vi "Group_Project-REV7.vi"() -> ()   [LabVIEW 2022 SP3]
uses:
  Control 1.ctl
panel:
  out "Train Waiting":bool=TRUE
  out "Boolean":bool=TRUE
  out "Numeric":i32
  out "Train go which way":dbl
  out "Increment Slider":bool=TRUE
  out "Timestamp for slide":i32
  out "Time stamp for wait":i32
  out "Ready for train":bool
  out "Train Progress":dbl(slide) scale=0.0..100.0
  out "Train Nearby Sensor 2":bool
  out "Train Nearby Sensor 1":bool
  out "Wait Time":i32
  out "Traffic Count":i32
  out "Observe traffic":bool
  out "Busy traffic":bool
  out "Add wait time":i32
  out "Numeric 5":u32
  out "Cars to Stop":bool
  out "Numeric 4":u32
  out "Car To Go":bool
  out "Train?":bool
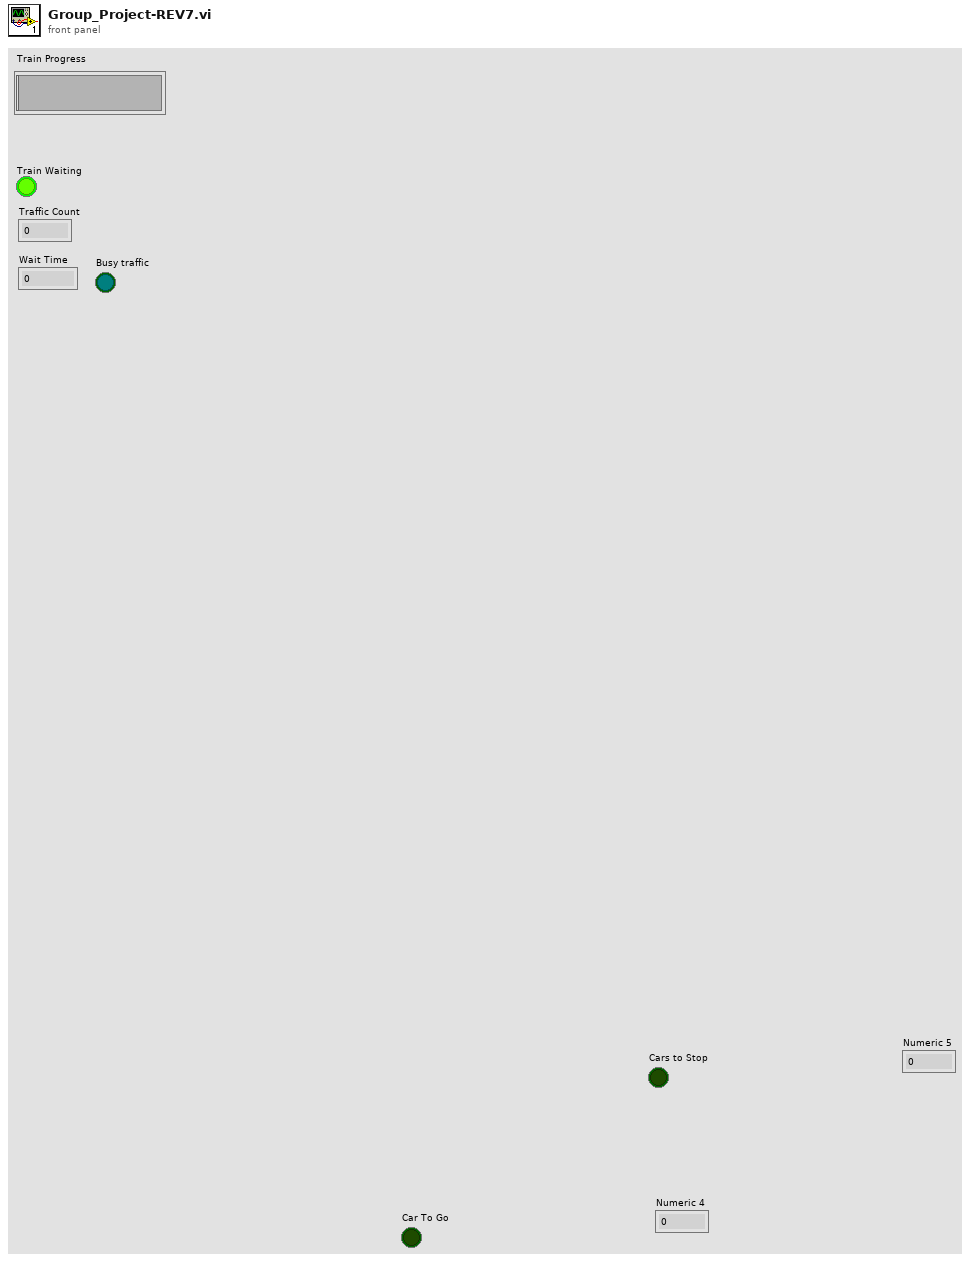
[diagram p1: front panel]
types:
  T1 = typedef "Control 1.ctl" = enum16{"None", "Down", "Up"}
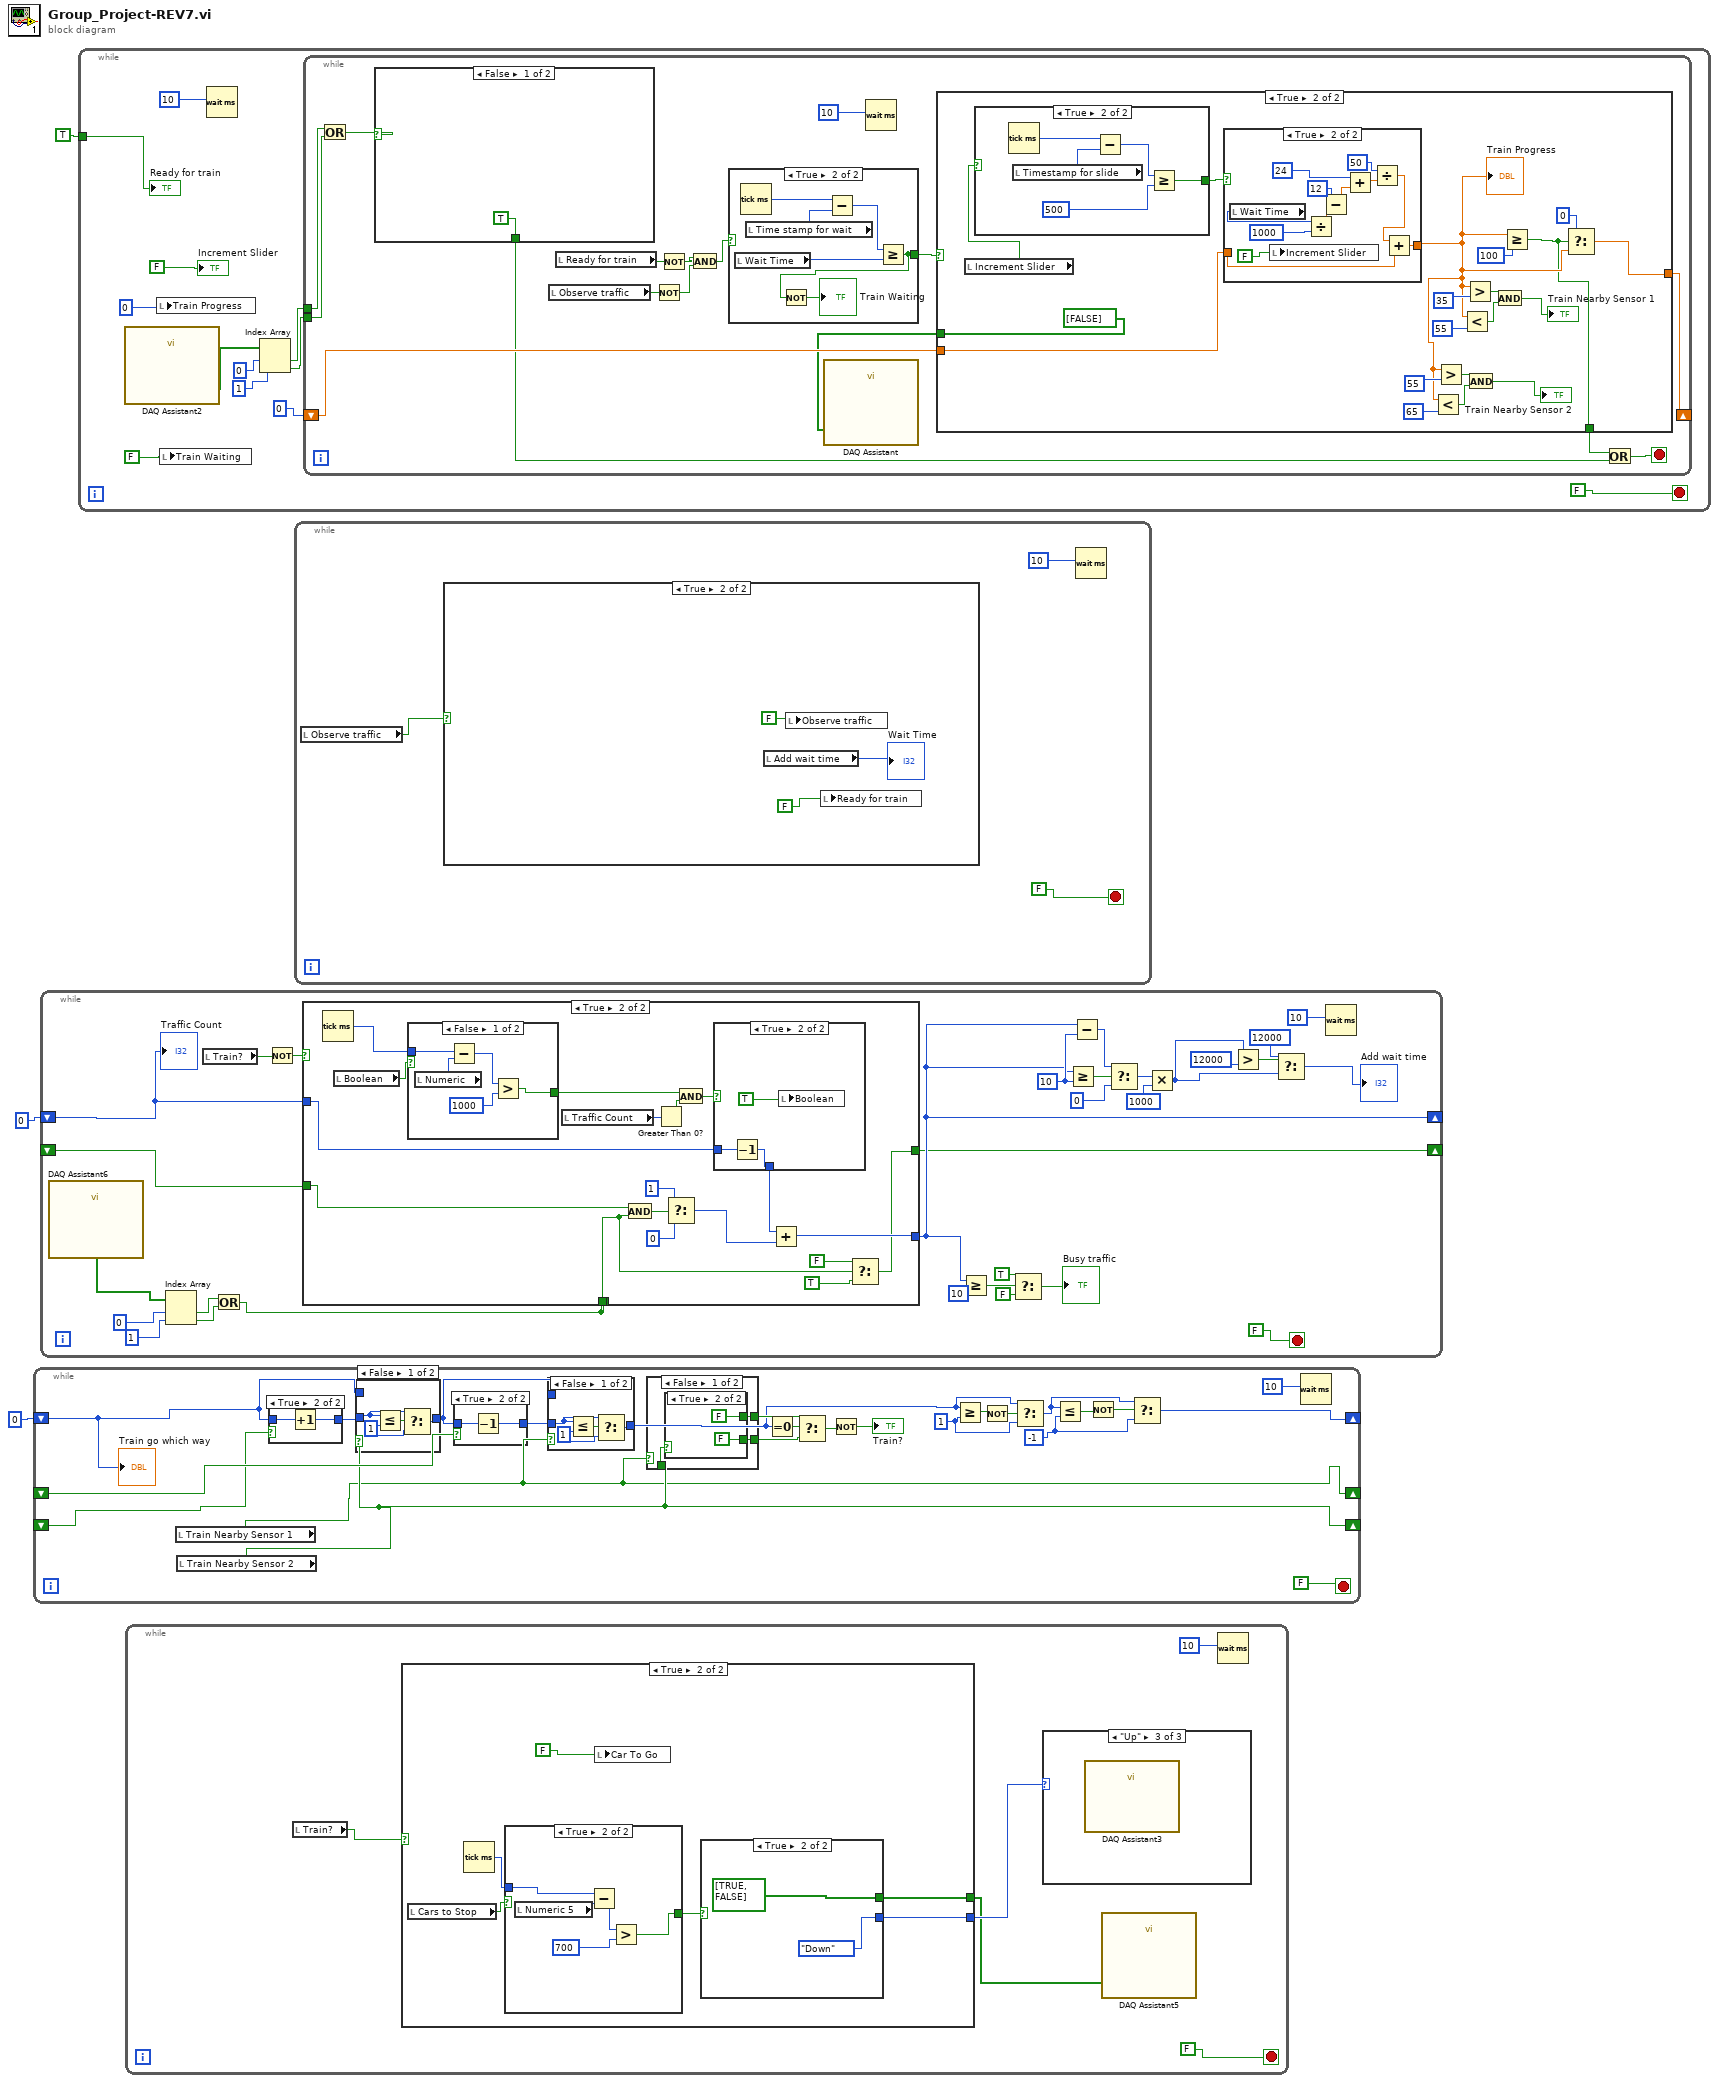
[diagram p0: block diagram]
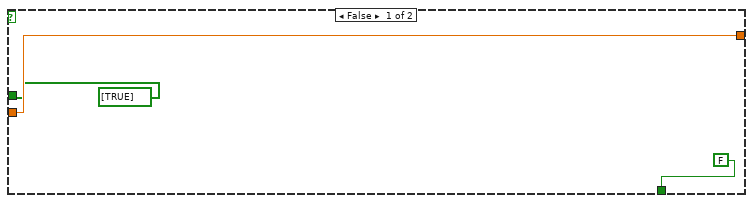
[diagram p3: hidden frame]
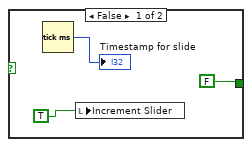
[diagram p5: hidden frame]
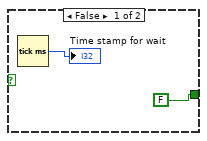
[diagram p6: hidden frame]
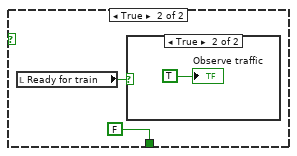
[diagram p7: hidden frame]
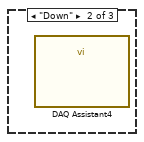
[diagram p10: hidden frame]
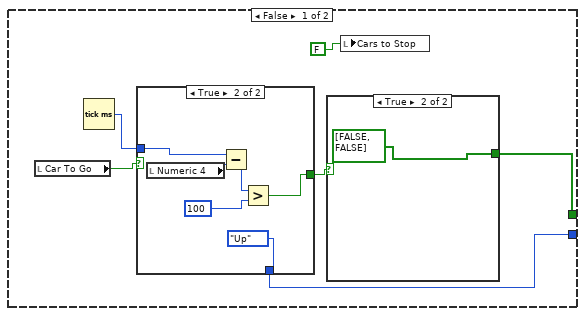
[diagram p11: hidden frame]
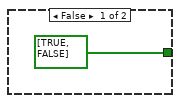
[diagram p12: hidden frame]
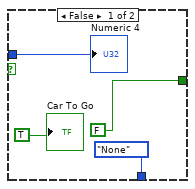
[diagram p13: hidden frame]
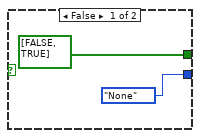
[diagram p14: hidden frame]
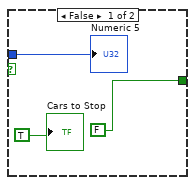
[diagram p15: hidden frame]
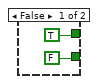
[diagram p16: hidden frame]
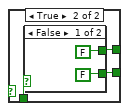
[diagram p17: hidden frame]
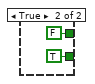
[diagram p18: hidden frame]
diagram:
  n1 = while {
    shift-right: [w8] -> _
    shift-left: 0 -> [w4]
    shift-right: [w6] -> _
    shift-left: _ -> [w10]
    shift-right: [w5] -> _
    shift-left: _ -> [w11]
    stop <- FALSE stop-if-true
    w14 = -1
    w17 = 1
    n2 = local read "Train Nearby Sensor 1"() -> (w5:bool)
    n3 = local read "Train Nearby Sensor 2"() -> (w6:bool)
    n4 = case shown="True" w10 {
      tunnel: [w55 w57] -> w27
      tunnel: w4 -> [w55 w56]
      frame False {
      }
      frame True {
        n5 = Increment(x=w56) -> (x+1=w57:i32)
      }
    }
    n6 = case shown="False" w6 {
      tunnel: w27 -> [w52 _]
      tunnel: [w50 w54] -> w26
      tunnel: w4 -> [_ w54]
      frame False {
        w51 = 1
        n7 = Less Or Equal?(x=w52, y=w51) -> (x <= y?=w53:bool)
        n8 = Select(t=w52, s=w53, f=w51) -> (s? t:f=w50:i32)
      }
      frame True {
      }
    }
    n9 = case shown="True" w11 {
      tunnel: w26 -> [w47 w49]
      tunnel: [w47 w48] -> w25
      frame False {
      }
      frame True {
        n10 = Decrement(x=w49) -> (x-1=w48:i32)
      }
    }
    n11 = case shown="False" w5 {
      tunnel: w26 -> [_ w46]
      tunnel: w25 -> [w43 _]
      tunnel: [w42 w46] -> w18
      frame False {
        w44 = 1
        n12 = Less Or Equal?(x=w43, y=w44) -> (x <= y?=w45:bool)
        n13 = Select(t=w43, s=w45, f=w44) -> (s? t:f=w42:i32)
      }
      frame True {
      }
    }
    n14 = case shown="False" w5 {
      tunnel: w6 -> [w28 w37]
      tunnel: [w29 w35] -> w23
      tunnel: [w30 w36] -> w22
      frame False {
        n15 = case shown="True" w28 {
          tunnel: [TRUE FALSE] -> w29
          tunnel: [FALSE FALSE] -> w30
          frame False {
          }
          frame True {
          }
        }
      }
      frame True {
        n16 = case shown="False" w37 {
          tunnel: [FALSE FALSE] -> w35
          tunnel: [FALSE TRUE] -> w36
          frame False {
          }
          frame True {
          }
        }
      }
    }
    n17 = Equal To 0?(x=w18) -> (x = 0?=w24:bool)
    n18 = Select(t=w23, s=w24, f=w22) -> (s? t:f=w21:bool)
    n19 = Not(x=w21) -> (.not. x?=→"Train?":bool)
    n20 = Greater Or Equal?(x=w18, y=w17) -> (x >= y?=w19:bool)
    n21 = Not(x=w19) -> (.not. x?=w20:bool)
    n22 = Select(t=w18, s=w20, f=w17) -> (s? t:f=w13:i32)
    n23 = Less Or Equal?(x=w13, y=w14) -> (x <= y?=w16:bool)
    n24 = Not(x=w16) -> (.not. x?=w15:bool)
    n25 = Select(t=w13, s=w15, f=w14) -> (s? t:f=w8:i32)
    n26 = Wait (ms)(milliseconds to wait=10) -> ()  [unwired: 1 out]
    "Train go which way" <- w4
  }
  n27 = while {
    shift-right: [w60] -> _
    shift-left: 0 -> [w62]
    shift-right: [w59] -> _
    shift-left: _ -> [w61]
    stop <- FALSE stop-if-true
    w85 = 10
    n28 = call "DAQ Assistant6"() -> ("data"=w69:bool[])  [unwired: 17 in, 2 out]
    n29 = Index Array(array=w69, index #1=0, index #2=1) -> (element #1=w66:bool, element #2=w65:bool)
    n30 = local read "Train?"() -> (w64:bool)
    n31 = Or(x=w66, y=w65) -> (x .or. y?=w58:bool)
    n32 = Not(x=w64) -> (.not. x?=w63:bool)
    n33 = case shown="True" w63 {
      tunnel: w62 -> [w92 w110]
      tunnel: w61 -> [w88 w106]
      tunnel: [w91 w104] -> w60
      tunnel: [w90 w101] -> w59
      tunnel: w58 -> [w89 _]
      tunnel: w58 -> [_ w100]
      frame False {
        n34 = And(x=w88, y=w89) -> (x .and. y?=w98:bool)
        n35 = Select(t=1, s=w98, f=0) -> (s? t:f=w95:i32)
        n36 = Add(x=w92, y=w95) -> (x+y=w91:i32)
        n37 = Select(t=FALSE, s=w89, f=TRUE) -> (s? t:f=w90:bool)
      }
      frame True {
        n38 = Tick Count (ms)() -> (millisecond timer value=w116:u32)
        n39 = local read "Boolean"() -> (w115:bool)
        n40 = case shown="False" w115 {
          tunnel: w116 -> [w124 w127]
          tunnel: [w121 w126] -> w114
          frame False {
            n41 = local read "Numeric"() -> (w125:i32)
            n42 = Subtract(x=w124, y=w125) -> (x-y=w122:u32)
            n43 = Greater?(x=w122, y=1000) -> (0:w121:bool)
          }
          frame True {
            w126 = FALSE
            "Numeric" <- w127
            "Boolean" <- w126
          }
        }
        n44 = local read "Traffic Count"() -> (w113:i32)
        n45 = And(x=w106, y=w100) -> (x .and. y?=w109:bool)
        n46 = Greater Than 0?(x=w113) -> (x > 0?=w112:bool)
        n47 = Select(t=1, s=w109, f=0) -> (s? t:f=w105:i32)
        n48 = And(x=w114, y=w112) -> (x .and. y?=w111:bool)
        n49 = case shown="True" w111 {
          tunnel: w110 -> [w117 w119]
          tunnel: [w117 w120] -> w99
          frame False {
          }
          frame True {
            n50 = Decrement(x=w119) -> (x-1=w120:i32)
            n51 = local write "Boolean"(TRUE) -> ()
          }
        }
        n52 = Add(x=w99, y=w105) -> (x+y=w104:i32)
        n53 = Select(t=FALSE, s=w100, f=TRUE) -> (s? t:f=w101:bool)
      }
    }
    n54 = Greater Or Equal?(x=w60, y=10) -> (x >= y?=w79:bool)
    n55 = Select(t=TRUE, s=w79, f=FALSE) -> (s? t:f=→"Busy traffic":bool)
    n56 = Greater Or Equal?(x=w60, y=w85) -> (x >= y?=w86:bool)
    n57 = Subtract(x=w60, y=w85) -> (x-y=w84:i32)
    n58 = Select(t=w84, s=w86, f=0) -> (s? t:f=w82:i32)
    n59 = Multiply(x=w82, y=1000) -> (x*y=w72:i32)
    n60 = Greater?(x=w72, y=12000) -> (0:w73:bool)
    n61 = Select(t=12000, s=w73, f=w72) -> (s? t:f=→"Add wait time":i32)
    n62 = Wait (ms)(milliseconds to wait=10) -> ()  [unwired: 1 out]
    "Traffic Count" <- w62
  }
  n63 = while {
    tunnel: TRUE -> [w130]
    stop <- FALSE stop-if-true
    n64 = call "DAQ Assistant2"() -> ("data"=w135:bool[])  [unwired: 17 in, 2 out]
    n65 = local write "Train Progress"(0) -> ()
    n66 = local write "Train Waiting"(FALSE) -> ()
    n67 = Wait (ms)(milliseconds to wait=10) -> ()  [unwired: 1 out]
    n68 = Index Array(array=w135, index #1=0, index #2=1) -> (element #1=w132:bool, element #2=w131:bool)
    n69 = while {
      tunnel: w132 -> [w155]
      tunnel: w131 -> [w149]
      shift-right: [w147] -> _
      shift-left: 0 -> [w148]
      stop <- w142 stop-if-true
      n70 = Or(x=w155, y=w149) -> (x .or. y?=w154:bool)
      n71 = case shown="False" w154 {
        tunnel: [TRUE FALSE] -> w141
        frame False {
        }
        frame True {
          n72 = local read "Ready for train"() -> (w209:bool)
          n73 = case shown="True" w209 {
            frame False {
            }
            frame True {
              "Observe traffic" <- TRUE
            }
          }
        }
      }
      n74 = local read "Observe traffic"() -> (w153:bool)
      n75 = local read "Ready for train"() -> (w144:bool)
      n76 = Not(x=w153) -> (.not. x?=w152:bool)
      n77 = Not(x=w144) -> (.not. x?=w145:bool)
      n78 = And(x=w145, y=w152) -> (x .and. y?=w151:bool)
      n79 = case shown="True" w151 {
        tunnel: [FALSE w201] -> w150
        frame False {
          n80 = Tick Count (ms)() -> (millisecond timer value=→"Time stamp for wait":u32)
        }
        frame True {
          n81 = local read "Wait Time"() -> (w203:i32)
          n82 = Tick Count (ms)() -> (millisecond timer value=w205:u32)
          n83 = local read "Time stamp for wait"() -> (w206:i32)
          n84 = Subtract(x=w205, y=w206) -> (x-y=w204:u32)
          n85 = Greater Or Equal?(x=w204, y=w203) -> (x >= y?=w201:bool)
          n86 = Not(x=w201) -> (.not. x?=→"Train Waiting":bool)
        }
      }
      n87 = Wait (ms)(milliseconds to wait=10) -> ()  [unwired: 1 out]
      n88 = case shown="True" w150 {
        tunnel: w148 -> [w158 w175]
        tunnel: [w158 w164] -> w147
        tunnel: [FALSE w160] -> w143
        tunnel: [bool[] [TRUE] bool[] [FALSE]] -> w140
        frame False {
        }
        frame True {
          n89 = local read "Increment Slider"() -> (w177:bool)
          n90 = case shown="True" w177 {
            tunnel: [FALSE w194] -> w176
            frame False {
              n91 = Tick Count (ms)() -> (millisecond timer value=→"Timestamp for slide":u32)
              n92 = local write "Increment Slider"(TRUE) -> ()
            }
            frame True {
              n93 = Tick Count (ms)() -> (millisecond timer value=w198:u32)
              n94 = local read "Timestamp for slide"() -> (w197:i32)
              n95 = Subtract(x=w198, y=w197) -> (x-y=w196:u32)
              n96 = Greater Or Equal?(x=w196, y=500) -> (x >= y?=w194:bool)
            }
          }
          n97 = case shown="True" w176 {
            tunnel: w175 -> [w178 w184]
            tunnel: [w178 w183] -> w165
            frame False {
            }
            frame True {
              n98 = local read "Wait Time"() -> (w189:i32)
              n99 = local write "Increment Slider"(FALSE) -> ()
              n100 = Divide(x=w189, y=1000) -> (x/y=w181:dbl)
              n101 = Subtract(x=12, y=w181) -> (x-y=w179:dbl)
              n102 = Add(x=24, y=w179) -> (x+y=w186:dbl)
              n103 = Divide(x=50, y=w186) -> (x/y=w185:dbl)
              n104 = Add(x=w185, y=w184) -> (x+y=w183:dbl)
            }
          }
          "Train Progress" <- w165
          n105 = Less?(x=w165, y=65) -> (x < y?=w168:bool)
          n106 = Greater?(x=w165, y=55) -> (0:w169:bool)
          n107 = Less?(x=w165, y=55) -> (x < y?=w172:bool)
          n108 = Greater?(x=w165, y=35) -> (0:w173:bool)
          n109 = And(x=w169, y=w168) -> (x .and. y?=→"Train Nearby Sensor 2":bool)
          n110 = And(x=w173, y=w172) -> (x .and. y?=→"Train Nearby Sensor 1":bool)
          n111 = Greater Or Equal?(x=w165, y=100) -> (x >= y?=w160:bool)
          n112 = Select(t=0, s=w160, f=w165) -> (s? t:f=w164:dbl)
        }
      }
      n113 = call "DAQ Assistant"("data"=w140) -> ()  [unwired: 17 in, 2 out]
      n114 = Or(x=w143, y=w141) -> (x .or. y?=w142:bool)
    }
    "Increment Slider" <- FALSE
    "Ready for train" <- w130
  }
  n115 = while {
    stop <- FALSE stop-if-true
    n116 = local read "Train?"() -> (w214:bool)
    n117 = case shown="True" w214 {
      tunnel: [w218 w236] -> w211
      tunnel: [w216 w234] -> w215
      frame False {
        n118 = local read "Car To Go"() -> (w221:bool)
        n119 = Tick Count (ms)() -> (millisecond timer value=w219:u32)
        n120 = case shown="True" w221 {
          tunnel: [FALSE w229] -> w220
          tunnel: w219 -> [w226 w233]
          tunnel: [Control_1."None" Control_1."Up"] -> w216
          frame False {
            "Numeric 4" <- w226
            "Car To Go" <- TRUE
          }
          frame True {
            n121 = local read "Numeric 4"() -> (w232:u32)
            n122 = Subtract(x=w233, y=w232) -> (x-y=w231:u32)
            n123 = Greater?(x=w231, y=100) -> (0:w229:bool)
          }
        }
        n124 = case shown="True" w220 {
          tunnel: [bool[] [TRUE, FALSE] bool[] [FALSE, FALSE]] -> w218
          frame False {
          }
          frame True {
          }
        }
        n125 = local write "Cars to Stop"(FALSE) -> ()
      }
      frame True {
        n126 = local read "Cars to Stop"() -> (w239:bool)
        n127 = Tick Count (ms)() -> (millisecond timer value=w237:u32)
        n128 = case shown="True" w239 {
          tunnel: [FALSE w247] -> w238
          tunnel: w237 -> [w245 w251]
          frame False {
            "Numeric 5" <- w245
            "Cars to Stop" <- TRUE
          }
          frame True {
            n129 = local read "Numeric 5"() -> (w250:u32)
            n130 = Subtract(x=w251, y=w250) -> (x-y=w249:u32)
            n131 = Greater?(x=w249, y=700) -> (0:w247:bool)
          }
        }
        n132 = local write "Car To Go"(FALSE) -> ()
        n133 = case shown="True" w238 {
          tunnel: [bool[] [FALSE, TRUE] bool[] [TRUE, FALSE]] -> w236
          tunnel: [Control_1."None" Control_1."Down"] -> w234
          frame False {
          }
          frame True {
          }
        }
      }
    }
    n134 = case shown="\"Up\"" w215 {
      frame "None", Default {
      }
      frame "Down" {
        n135 = call "DAQ Assistant4"() -> ()  [unwired: 18 in, 2 out]
      }
      frame "Up" {
        n136 = call "DAQ Assistant3"() -> ()  [unwired: 18 in, 2 out]
      }
    }
    n137 = call "DAQ Assistant5"("data"=w211) -> ()  [unwired: 17 in, 2 out]
    n138 = Wait (ms)(milliseconds to wait=10) -> ()  [unwired: 1 out]
  }
  n139 = while {
    stop <- FALSE stop-if-true
    n140 = local read "Observe traffic"() -> (w253:bool)
    n141 = case shown="True" w253 {
      frame False {
      }
      frame True {
        n142 = local read "Add wait time"() -> (→"Wait Time":i32)
        n143 = local write "Observe traffic"(FALSE) -> ()
        n144 = local write "Ready for train"(FALSE) -> ()
      }
    }
    n145 = Wait (ms)(milliseconds to wait=10) -> ()  [unwired: 1 out]
  }
